vi "OpenServerComm.vi"() -> (1 "Connected":bool, 2 "Quitted":bool=TRUE)   [LabVIEW 2014]
uses:
  globals/AzCamGlobals.vi
panel:
  out "Message":string
  in  "Connect":bool
  in  "Server Port":u16=2402
  in  "Server Name":string="ccd"
  in  "Quit":bool
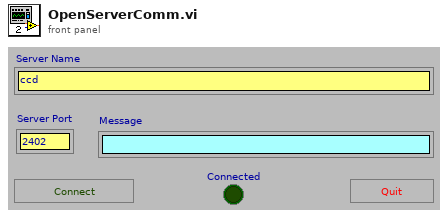
[diagram p1: front panel]
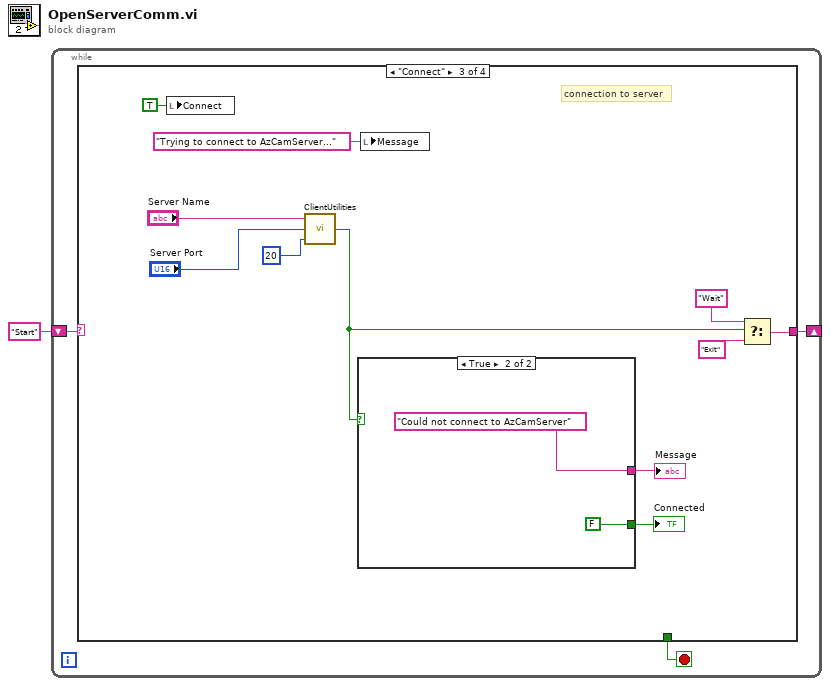
[diagram p0: block diagram]
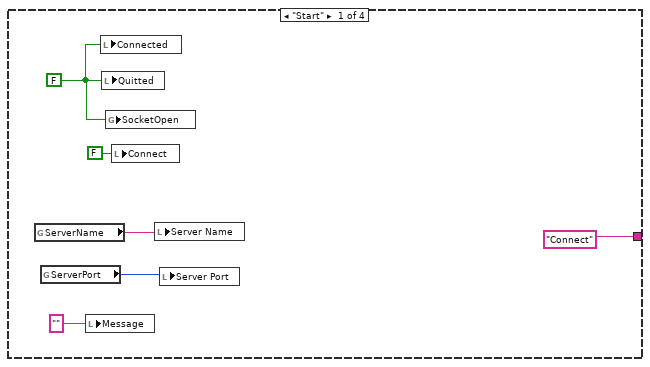
[diagram p2: hidden frame]
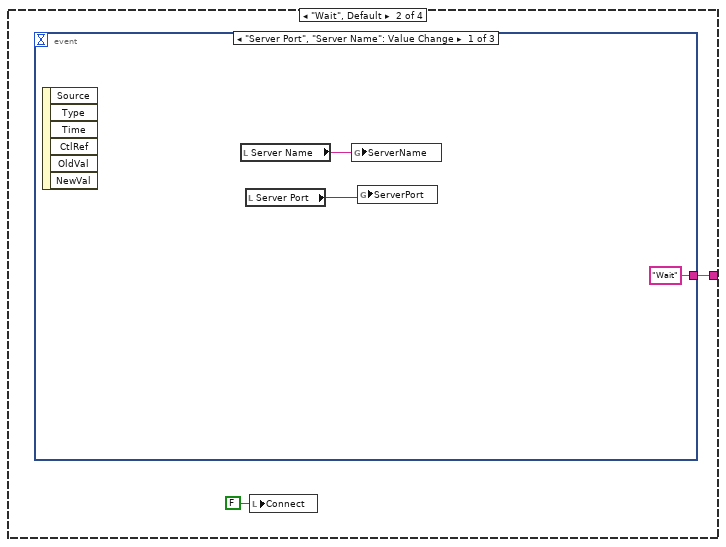
[diagram p3: hidden frame]
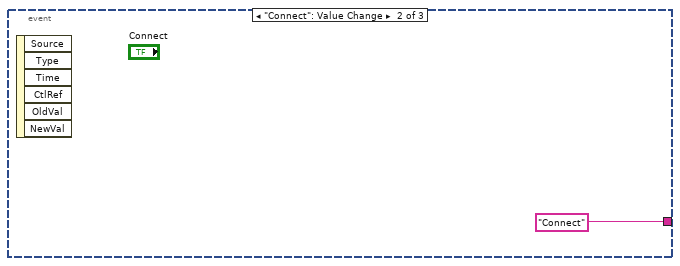
[diagram p4: hidden frame]
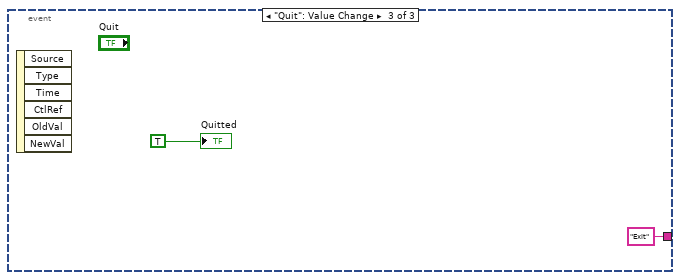
[diagram p5: hidden frame]
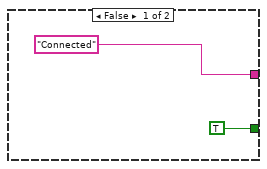
[diagram p6: hidden frame]
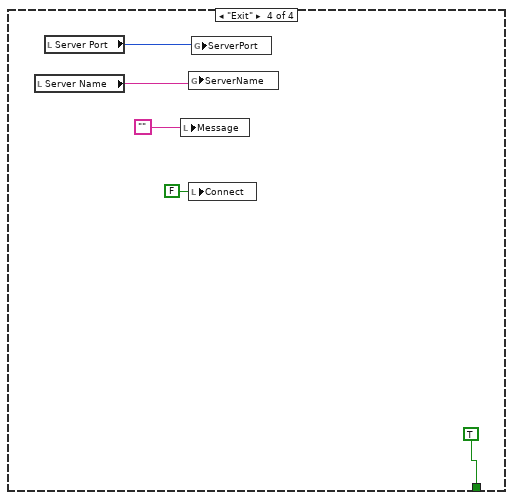
[diagram p7: hidden frame]
diagram:
  n1 = while {
    shift-right: [w2] -> _
    shift-left: "Start" -> [w3]
    stop <- w4 stop-if-true
    n2 = case shown="\"Connect\"" w3 {
      tunnel: [_ _ _ TRUE] -> w4
      tunnel: ["Connect" w12 w29 _] -> w2
      frame "Start" {
        w7 = FALSE ("Quitted")
        n3 = global read "AzCamGlobals.vi" "ServerName"() -> (w9:string)
        n4 = global read "AzCamGlobals.vi" "ServerPort"() -> (w10:i32)
        n5 = local write "Message"("" ("Message")) -> ()
        n6 = local write "Connected"(w7) -> ()
        n7 = local write "Quitted"(w7) -> ()
        n8 = global write "AzCamGlobals.vi" "SocketOpen"(w7) -> ()
        n9 = local write "Connect"(FALSE ("Connect")) -> ()
        n10 = local write "Server Name"(w9) -> ()
        n11 = local write "Server Port"(w10) -> ()
      }
      frame "Wait", Default {
        n12 = event shown="[0] \"Server Port\", \"Server Name\": Value Change" {
          selector: _ -> [_ _ _]
          dyn-events: _ -> [_ _ _]
          timeout: _ -> [_ _ _]
          tunnel: ["Wait" "Connect" "Exit"] -> w12
          event "Server Port", "Server Name": Value Change {
            n13 = event-data() -> ()  [unwired: 1 in, 6 out]
            n14 = local read "Server Name"() -> (w14:string)
            n15 = local read "Server Port"() -> (w13:u16)
            n16 = global write "AzCamGlobals.vi" "ServerName"(w14) -> ()
            n17 = global write "AzCamGlobals.vi" "ServerPort"(w13) -> ()
          }
          event "Connect": Value Change {
            n18 = event-data() -> ()  [unwired: 1 in, 6 out]
          }
          event "Quit": Value Change {
            n19 = event-data() -> ()  [unwired: 1 in, 6 out]
            "Quitted" <- TRUE ("Quitted")
          }
        }
        n20 = local write "Connect"(FALSE ("Connect")) -> ()
      }
      frame "Connect" {
        # "connection to server"
        n21 = local write "Connect"(TRUE ("Connect")) -> ()
        n22 = call "ClientUtilities.vi"("Timout"=u8 20, "ServerPort"="Server Port", "ServerName"="Server Name") -> ("Error"=w20:bool)
        n23 = case shown="True" w20 {
          tunnel: ["Connected" ("message") "Could not connect to AzCamServer" ("message")] -> w28
          tunnel: [TRUE ("Connected") FALSE ("Connected")] -> w27
          frame False {
          }
          frame True {
          }
        }
        "Message" <- w28
        "Connected" <- w27
        n24 = local write "Message"("Trying to connect to AzCamServer..." ("Message")) -> ()
        n25 = Select(t="Wait", s=w20, f="Exit") -> (s? t:f=w29:string)
      }
      frame "Exit" {
        n26 = local read "Server Name"() -> (w37:string)
        n27 = local read "Server Port"() -> (w36:u16)
        n28 = local write "Message"("") -> ()
        n29 = global write "AzCamGlobals.vi" "ServerName"(w37) -> ()
        n30 = local write "Connect"(FALSE ("Connect")) -> ()
        n31 = global write "AzCamGlobals.vi" "ServerPort"(w36) -> ()
      }
    }
  }
